vi "Get Depth Frame.vi"(8 "error in (no error)":errorcluster, 11 "Kinect Session in":refnum<class "Kinect Session.lvclass">) -> (0 "error out":errorcluster, 2 "Depth Frame":T1(plugin-control), 3 "Kinect Session out":refnum<class "Kinect Session.lvclass">)   [LabVIEW 2014, in "Kinect Library.lvlib"]
doc: "This VI will retrieve the latest depth image. If this function is called too frequently, it can return an error. If the function is called too sparsely, nothing bad will happen."
uses:
  Kinect Library.lvlib
  Kinect Session Class/Kinect Session.lvclass
  Microsoft.Kinect
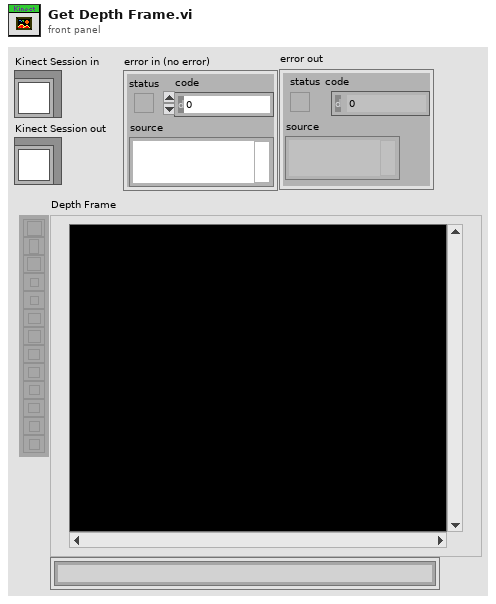
[diagram p1: front panel]
types:
  T1 = typedef "IMAQ Image.ctl" = refnum<image>
  T2 = cluster{"FramePixelDataLength":i32, "FrameWidth":i32, "FrameHeight":i32}
  T3 = cluster{"status":bool, "code":bool, "source":bool}
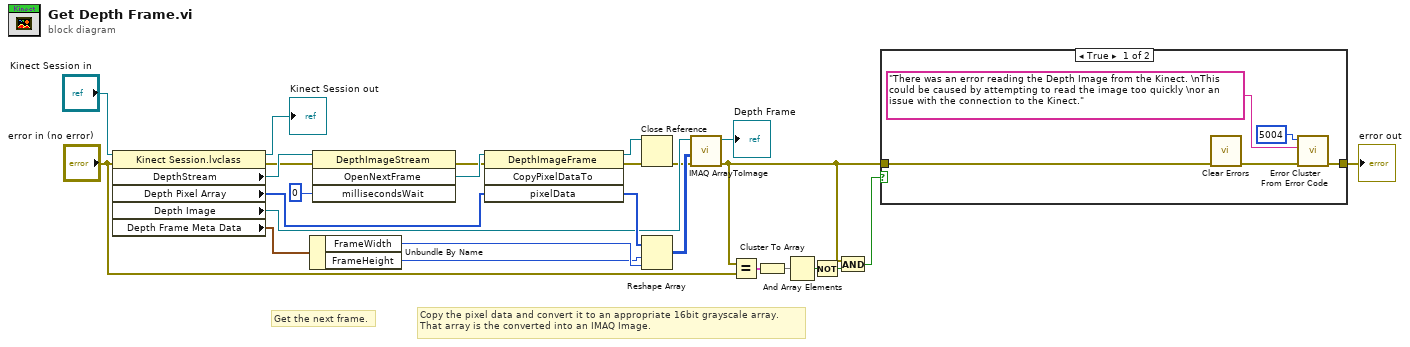
[diagram p0: block diagram]
diagram:
  # "Copy the pixel data and convert it to an appropriate 16bit grayscale array.\nThat array is the converted into an IMAQ Image."
  # "Get the next frame."
  n1 = property class="Kinect Session.lvclass"(reference="Kinect Session in", error in="error in (no error)") -> (reference out=→"Kinect Session out":refnum<class "Kinect Session.lvclass">, error out=w13:errorcluster, "DepthStream"=w24:refnum<k24>, "Depth Pixel Array"=w21:i16[], "Depth Image"=w12:T1, "Depth Frame Meta Data"=w19:T2)
  n2 = Unbundle By Name(w19) -> ("FrameWidth"=w18:i32, "FrameHeight"=w17:i32)
  n3 = invoke class="DepthImageStream" method="OpenNextFrame"(reference=w24, error in=w13, "millisecondsWait"=0) -> (error out=w15:errorcluster, "OpenNextFrame"=w22:refnum<k24>)  [unwired: 1 in, 2 out]
  n4 = invoke class="DepthImageFrame" method="CopyPixelDataTo"(reference=w22, error in=w15, "pixelData"=w21) -> (reference out=w16:refnum<k24>, error out=w14:errorcluster, "pixelData"=w20:i16[])  [unwired: 1 in, 1 out]
  n5 = Close Reference(reference=w16, error in (no error)=w14) -> (error out=w10:errorcluster)
  n6 = Reshape Array(w20, w17, w18) -> (w11:i16[][])
  n7 = call "IMAQ ArrayToImage"("error in (no error)"=w10, "Image Pixels (I16)"=w11, "Image"=w12) -> ("error out"=w4:errorcluster, "Image Out"=→"Depth Frame":T1)  [unwired: 7 in]
  n8 = Equal?(x=w4, y="error in (no error)") -> (x = y?=w8:T3)
  n9 = Cluster To Array(cluster=w8) -> (array=w7:bool[])
  n10 = And Array Elements(Boolean array=w7) -> (logical AND=w1:bool)
  n11 = Not(x=w1) -> (.not. x?=w6:bool)
  n12 = And(x=w4, y=w6) -> (x .and. y?=w3:bool)
  n13 = case shown="True" w3 {
    tunnel: [w31 w32] -> w5
    tunnel: w4 -> [w28 w32]
    frame True {
      n14 = call <vilib>:"Clear Errors.vi"("error in (no error)"=w28) -> ("error out"=w27:errorcluster)  [unwired: 5 in, 1 out]
      n15 = call <vilib>:"Error Cluster From Error Code.vi"("error in (no error)"=w27, "error message (\"\")"="There was an error reading the Depth Image from the Kinect. \nThis could be caused by attempting to read the image too quickly \nor an issue with the connection to the Kinect." ("error message (\"\")"), "error code (0)"=5004) -> ("error out"=w31:errorcluster)  [unwired: 6 in]
    }
    frame False {
    }
  }
  "error out" <- w5
